vi "aula 5.vi"() -> ()   [LabVIEW 2024]
uses:
  <vilib>/LabVIEW Open Source Project/Epoch Date & Time/epoch.UNIX/Epoch.UNIX.lvclass
panel:
  in  "Tab Control":T1(tab)
  out "Waveform Chart":waveform(dbl)(graph)
  out "Waveform Chart 2":waveform(dbl)(graph)
  out "Waveform Chart 3":waveform(dbl)(graph)
  out "Waveform Chart 4":waveform(dbl)(graph)
  in  "stop 4":bool
  in  "stop 3":bool
  in  "stop 2":bool
  in  "stop":bool
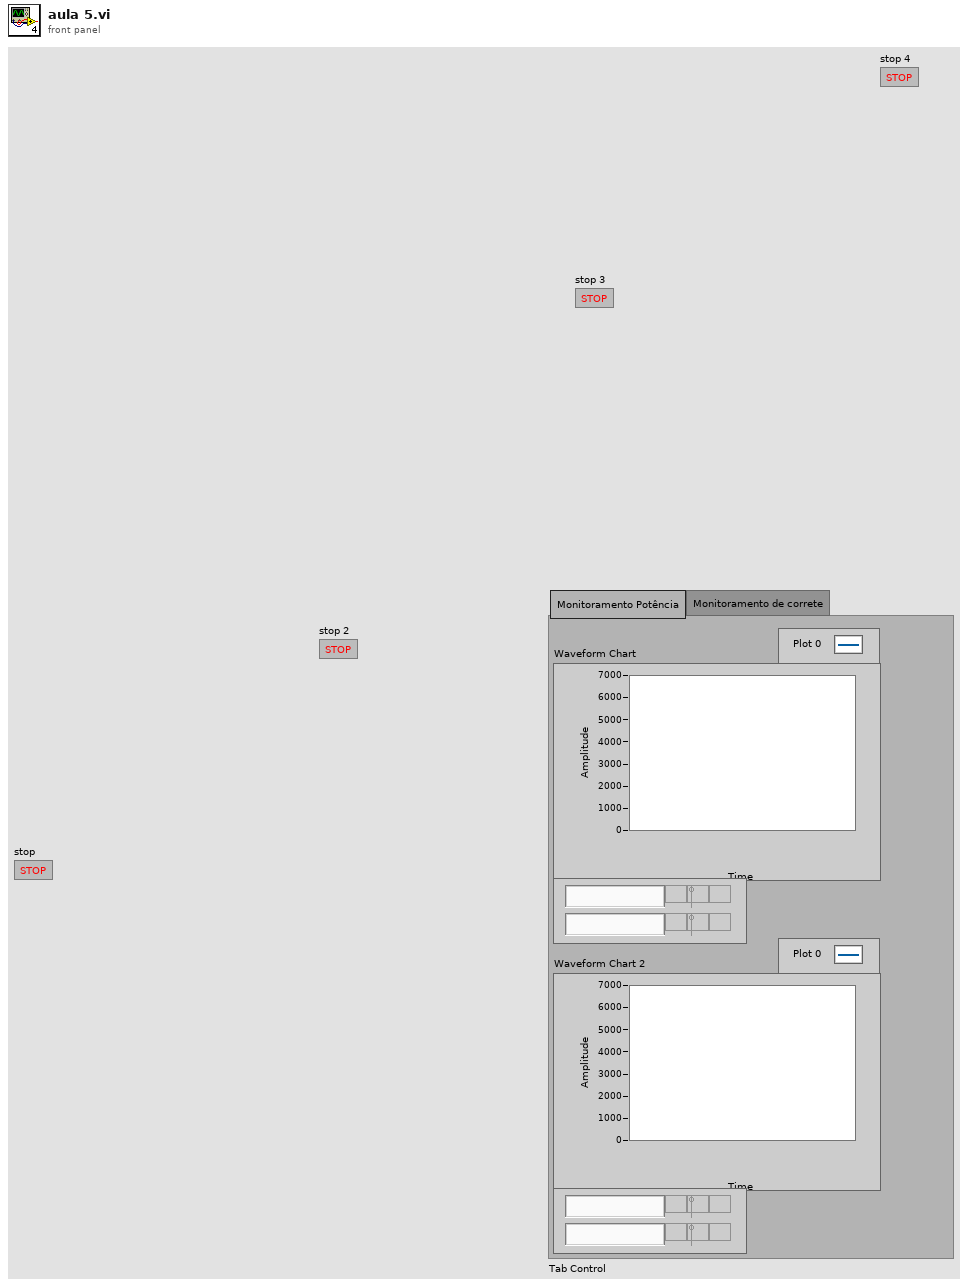
[diagram p1: front panel]
types:
  T1 = enum32{"Monitoramento Potência", "Monitoramento de correte"}
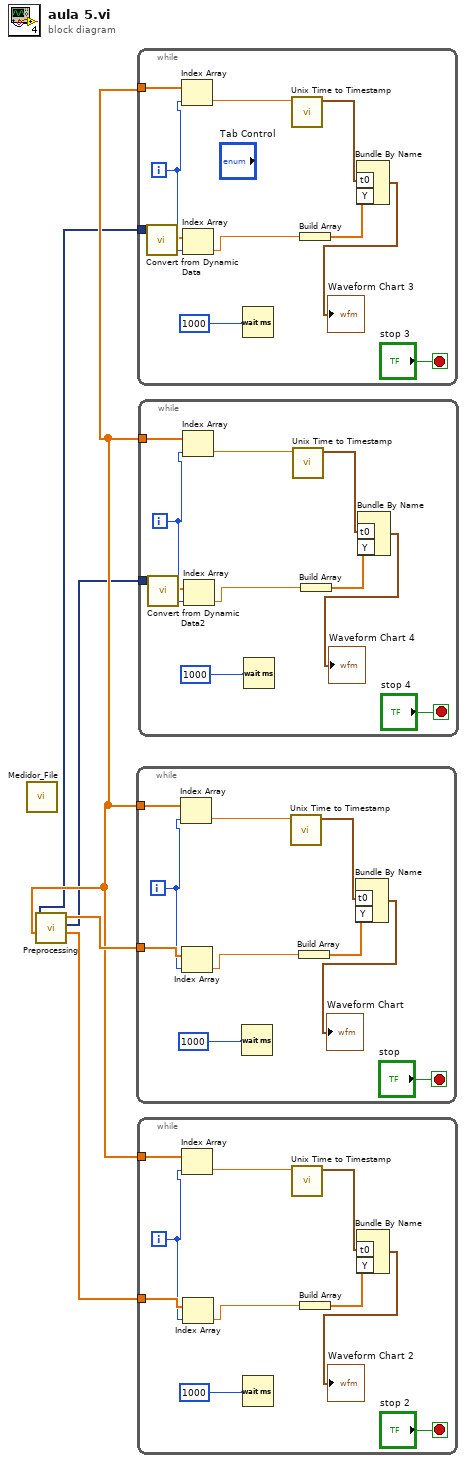
[diagram p0: block diagram]
diagram:
  n1 = call "Medidor_File.vi"() -> ()  [unwired: 7 out]
  n2 = call "Preprocessing.vi"() -> ("Potência Ativa B"=w4:dbl[], "Corrente C"=w1:dynamicdata, "Potência instantänea A"=w5:dbl[], "Timestamp"=w3:dbl[], "Corrente A"=w2:dynamicdata)  [unwired: 5 out]
  n3 = while {
    tunnel: w3 -> [w15]
    tunnel: w5 -> [w13]
    i -> [w12]
    stop <- "stop" stop-if-true
    n4 = Index Array(array=w15, index=w12) -> (element=w14:dbl)
    n5 = Index Array(array=w13, index=w12) -> (element=w10:dbl)
    n6 = Wait (ms)(milliseconds to wait=u32 1000) -> ()  [unwired: 1 out]
    n7 = call <vilib>:"Unix Time to Timestamp.vi"("Unix Time (s)"=w14) -> ("Timestamp"=w11:timestamp)  [unwired: 9 in, 1 out]
    n8 = Build Array(w10) -> (w9:dbl[])
    n9 = Bundle By Name("t0"=w11, "Y"=w9) -> (→"Waveform Chart":waveform(dbl))  [unwired: 1 in]
  }
  n10 = while {
    tunnel: w3 -> [w26]
    tunnel: w2 -> [w24]
    i -> [w23]
    stop <- "stop 3" stop-if-true
    n11 = call "Convert from Dynamic Data"("Dynamic Data Type"=w24) -> ("Array"=w16:dbl[])  [unwired: 3 in]
    n12 = Index Array(array=w26, index=w23) -> (element=w25:dbl)
    n13 = Index Array(array=w16, index=w23) -> (element=w21:dbl)
    n14 = Wait (ms)(milliseconds to wait=u32 1000) -> ()  [unwired: 1 out]
    n15 = call <vilib>:"Unix Time to Timestamp.vi"("Unix Time (s)"=w25) -> ("Timestamp"=w22:timestamp)  [unwired: 9 in, 1 out]
    n16 = Build Array(w21) -> (w20:dbl[])
    n17 = Bundle By Name("t0"=w22, "Y"=w20) -> (→"Waveform Chart 3":waveform(dbl))  [unwired: 1 in]
  }
  n18 = while {
    tunnel: w3 -> [w36]
    tunnel: w4 -> [w34]
    i -> [w33]
    stop <- "stop 2" stop-if-true
    n19 = Index Array(array=w36, index=w33) -> (element=w35:dbl)
    n20 = Index Array(array=w34, index=w33) -> (element=w31:dbl)
    n21 = Wait (ms)(milliseconds to wait=u32 1000) -> ()  [unwired: 1 out]
    n22 = call <vilib>:"Unix Time to Timestamp.vi"("Unix Time (s)"=w35) -> ("Timestamp"=w32:timestamp)  [unwired: 9 in, 1 out]
    n23 = Build Array(w31) -> (w30:dbl[])
    n24 = Bundle By Name("t0"=w32, "Y"=w30) -> (→"Waveform Chart 2":waveform(dbl))  [unwired: 1 in]
  }
  n25 = while {
    tunnel: w3 -> [w47]
    tunnel: w1 -> [w45]
    i -> [w44]
    stop <- "stop 4" stop-if-true
    n26 = call "Convert from Dynamic Data2"("Dynamic Data Type"=w45) -> ("Array"=w37:dbl[])  [unwired: 3 in]
    n27 = Index Array(array=w47, index=w44) -> (element=w46:dbl)
    n28 = Index Array(array=w37, index=w44) -> (element=w42:dbl)
    n29 = Wait (ms)(milliseconds to wait=u32 1000) -> ()  [unwired: 1 out]
    n30 = call <vilib>:"Unix Time to Timestamp.vi"("Unix Time (s)"=w46) -> ("Timestamp"=w43:timestamp)  [unwired: 9 in, 1 out]
    n31 = Build Array(w42) -> (w41:dbl[])
    n32 = Bundle By Name("t0"=w43, "Y"=w41) -> (→"Waveform Chart 4":waveform(dbl))  [unwired: 1 in]
  }
